vi "Inline Write (Interactions).vi"(8 "error in":errorcluster, 11 "RT State Variables in":T1 {"runtime data"."out object status BD"."Data Reference" format="%.0x"; "runtime data"."out object data BD"."Data Reference" format="%.0x"; "runtime data"."out interaction status BD"."Data Reference" format="%.0x"; "runtime data"."out interaction data BD"."Data Reference" format="%.0x"; "Settings"."objectData"."out object status BD"."Data Reference" format="%.0x"; "Settings"."objectData"."out object data BD"."Data Reference" format="%.0x"; "Settings"."objectData"."out interaction status BD"."Data Reference" format="%.0x"; "Settings"."objectData"."out interaction data BD"."Data Reference" format="%.0x"}) -> (0 "error out":errorcluster, 3 "RT State Variables out":T1 {"runtime data"."out object status BD"."Data Reference" format="%.0x"; "runtime data"."out object data BD"."Data Reference" format="%.0x"; "runtime data"."out interaction status BD"."Data Reference" format="%.0x"; "runtime data"."out interaction data BD"."Data Reference" format="%.0x"; "Settings"."objectData"."out object status BD"."Data Reference" format="%.0x"; "Settings"."objectData"."out object data BD"."Data Reference" format="%.0x"; "Settings"."objectData"."out interaction status BD"."Data Reference" format="%.0x"; "Settings"."objectData"."out interaction data BD"."Data Reference" format="%.0x"})   [LabVIEW 2019, in "HLA Custom Device Engine.lvlib"]
uses:
  HLA Custom Device Engine.lvlib
  RTStateVariables.ctl
  <vilib>/NI/NIVS Inline Async API/_VS Inline Async API/VS Inline Async API/VS Inline Async API.lvclass
  Shared/Compiled.Settings.ctl
  Shared/main_page_config.ctl
  Shared/object_managament_config.ctl
  Shared/interaction_parameter_configuration.ctl
  Shared/object_attribute_configuration.ctl
  Shared/object_status_info.ctl
  Shared/object_data.ctl
  <vilib>/NI VeriStand/Custom Device API/Block Data Reference.ctl
  <vilib>/NI VeriStand/Custom Device API/Data Reference.ctl
  RTruntimeData.ctl
  _typedefs/RThlaMapHelpers.ctl
  _typedefs/map_in_interaction.ctl
  _typedefs/map_interaction_value.ctl
  _typedefs/map_attr_param_data.ctl
  _typedefs/map_object.ctl
  _typedefs/map_object_key.ctl
  _typedefs/map_object_value.ctl
  _typedefs/map_object_instance.ctl
  _typedefs/map_object_instance_value.ctl
  _typedefs/map_object_vs_instance.ctl
  _typedefs/map_out_vs_ch_instanceId.ctl
  _typedefs/map_out_vs_ch_objects.ctl
  _typedefs/map_out_vs_ch_objects_value.ctl
  _typedefs/map_out_vs_ch_interactIonClass.ctl
  <vilib>/addons/hla/receiveInteractionEvent_type.ctl
  <vilib>/addons/hla/OrderType.ctl
  <vilib>/addons/hla/TransportationType.ctl
  <vilib>/addons/hla/reflectAttributeValuesEvent_type.ctl
  <vilib>/addons/hla/discoverObjectInstanceEvent_type.ctl
  <vilib>/addons/hla/removeObjectInstanceEvent_type.ctl
  <vilib>/NI VeriStand/Custom Device API/Global Data Refs.vi
  Data Encoding_Decoding/Set HLAfloat64BE.vi
  Data Encoding_Decoding/custom/Set fixed_coords.vi
  <vilib>/NI VeriStand/Custom Device API/Custom Device API.lvlib
  <vilib>/addons/hla/openrti_rti1516eLv.lvlib
  <vilib>/addons/hla/helpers/phvm.lvlib
  _Debug/VsDebugLibrary.lvlib
  Shared/HLA Custom Device Shared.lvlib
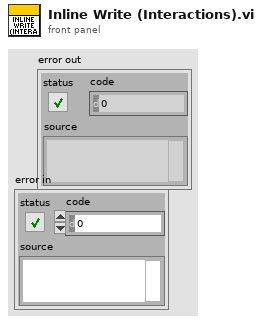
[diagram p1: front panel]
types:
  T1 = typedef "HLA Custom Device Engine.lvlib/RTStateVariables.ctl" = cluster{"Async":refnum<class "VS Inline Async API.lvclass">, "Settings":T2, "runtime data":T11}
  T2 = typedef "HLA Custom Device Shared.lvlib/Compiled.Settings.ctl" = cluster{"Name":string, "Async Init Timeout":u16, "main page properties":T3, "obiectConfig":T4, "objectStatus":T7, "objectData":T8}
  T3 = typedef "HLA Custom Device Shared.lvlib/main_page_config.ctl" = cluster{"Federate Execution Name":string, "Federate Type":string, "Local Designator Settings":string, "FOM Module":path, "mak mtl file":path, "FOM destination path":string, "MTL destination path":string}
  T4 = typedef "HLA Custom Device Shared.lvlib/object_managament_config.ctl" = cluster{"incoming interactions":T5[], "incoming objects":T6[], "outgoing interactions":T5[], "outgoing objects":T6[]}
  T5 = typedef "HLA Custom Device Shared.lvlib/interaction_parameter_configuration.ctl" = cluster{"interaction class name":string, "parameter name":string, "datatype":string, "vsChIndex":i32, "vsObjectId":string}
  T6 = typedef "HLA Custom Device Shared.lvlib/object_attribute_configuration.ctl" = cluster{"object class name":string, "instanceId":i32, "attribute name":string, "datatype":string, "vsChIndex":i32, "vsObjectId":string}
  T7 = typedef "HLA Custom Device Shared.lvlib/object_status_info.ctl" = cluster{"incoming interactions":map{string, map{string, i32}}, "incoming objects":map{string, map{string, i32}}, "outgoing interactions":map{string, map{string, i32}}, "outgoing objects":map{string, map{string, i32}}}
  T8 = typedef "HLA Custom Device Shared.lvlib/object_data.ctl" = cluster{"out interaction data BD":T9[], "out interaction data size":i32, "out interaction status BD":T9[], "out interaction status size":i32, "out object data BD":T9[], "out object data size":i32, "out object status BD":T9[], "out object status size":i32}
  T9 = typedef "Custom Device API.lvlib/Block Data Reference.ctl" = cluster{"Data Reference":T10, "Offset":u64, "Length":u64}
  T10 = typedef "Custom Device API.lvlib/Data Reference.ctl" = i32
  T11 = typedef "HLA Custom Device Engine.lvlib/RTruntimeData.ctl" = cluster{"rtiHandle":i64, "hlaMap":T12, "hla event registration":refnum<event-registration>, "out interaction data BD":T9[], "out interaction data":dbl[], "out interaction status BD":T9[], "out interaction status ":dbl[], "out object data BD":T9[], "out object data":dbl[], "out object status BD":T9[], "out object status ":dbl[]}
  T12 = typedef "HLA Custom Device Engine.lvlib/RThlaMapHelpers.ctl" = cluster{"in_interactionMap":T13, "in_objectMap":T16, "in_map_object_instance":T19, "in_map_vs_incoming_instance":T21, "out_map_vs_ch_instanceId":T22, "out_interactionMap":T13, "out_map_vs_ch_objectInstance":T23, "out_objectMap":T16, "out_map_vs_ch_interactionClass":T25}
  T13 = typedef "HLA Custom Device Engine.lvlib/map_in_interaction.ctl" = map{u64, T14}
  T14 = typedef "HLA Custom Device Engine.lvlib/map_interaction_value.ctl" = cluster{"infoChMap":map{string, i32}, "parameterMap":map{u64, T15}, "parHandleValueMap":u64}
  T15 = typedef "HLA Custom Device Engine.lvlib/map_attr_param_data.ctl" = cluster{"dataType":string, "offset":i32, "numOfElements":i32}
  T16 = typedef "HLA Custom Device Engine.lvlib/map_object.ctl" = map{T17, T18}
  T17 = typedef "HLA Custom Device Engine.lvlib/map_object_key.ctl" = cluster{"instanceId":i32, "objectClassHandle":u64}
  T18 = typedef "HLA Custom Device Engine.lvlib/map_object_value.ctl" = cluster{"infoChMap":map{string, i32}, "attributeMap":map{u64, T15}, "attrHandleSet":u64, "attrHandleValueMap":u64, "objectInstancePrefix":string}
  T19 = typedef "HLA Custom Device Engine.lvlib/map_object_instance.ctl" = map{u64, T20}
  T20 = typedef "HLA Custom Device Engine.lvlib/map_object_instance_value.ctl" = cluster{"objectClassHandle":u64, "objectInstanceName":string, "InstanceID":i32}
  T21 = typedef "HLA Custom Device Engine.lvlib/map_object_vs_instance.ctl" = map{u64, map{i32, u64}}
  T22 = typedef "HLA Custom Device Engine.lvlib/map_out_vs_ch_instanceId.ctl" = map{i32, i32}
  T23 = typedef "HLA Custom Device Engine.lvlib/map_out_vs_ch_objects.ctl" = map{i32, T24}
  T24 = typedef "HLA Custom Device Engine.lvlib/map_out_vs_ch_objects_value.ctl" = cluster{"objectInstanceHandle":u64, "objectClassHandle":u64}
  T25 = typedef "HLA Custom Device Engine.lvlib/map_out_vs_ch_interactIonClass.ctl" = map{i32, u64}
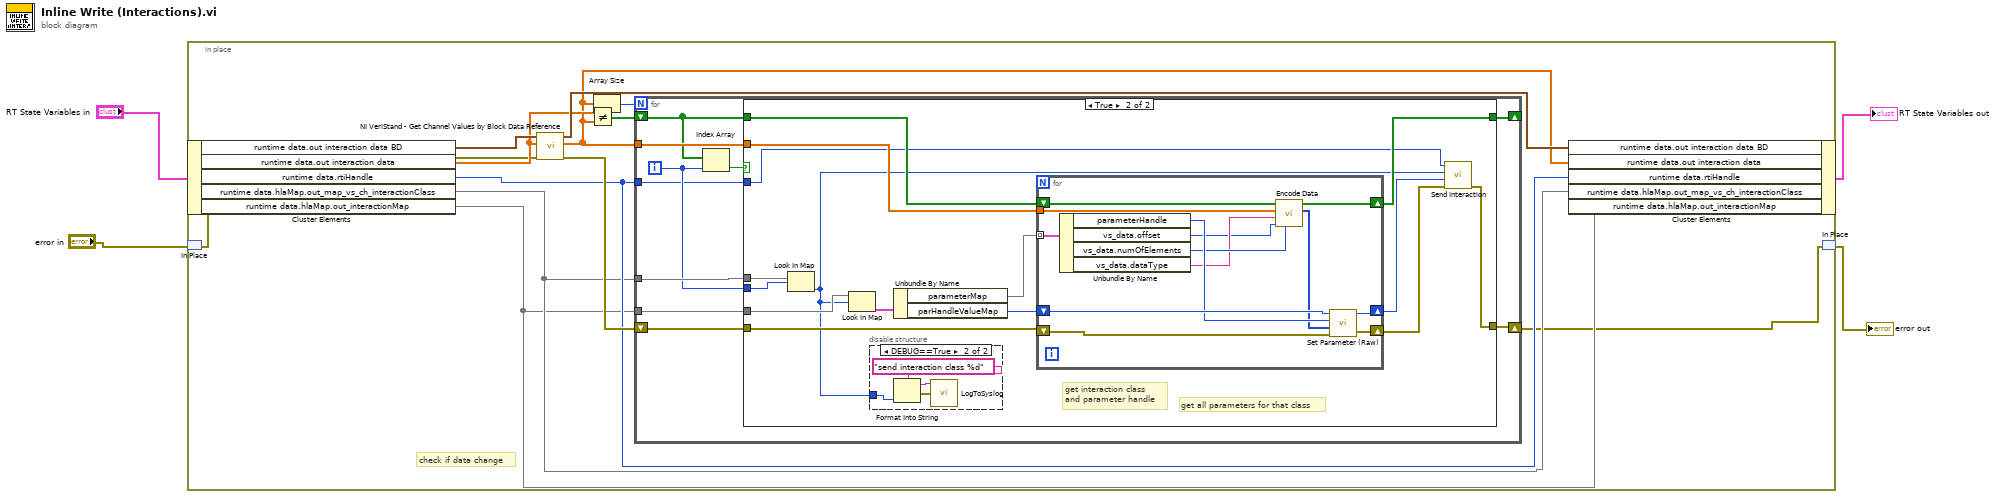
[diagram p0: block diagram]
diagram:
  n1 = in-place {
    # "check if data change"
    n2 = in-place-cluster #1("RT State Variables in") -> ("runtime data.out interaction data BD"=w16:T9[], "runtime data.out interaction data"=w8:dbl[], "runtime data.rtiHandle"=w11:i64, "runtime data.hlaMap.out_map_vs_ch_interactionClass"=w10:T25, "runtime data.hlaMap.out_interactionMap"=w9:T13)
    n3 = in-place-match #2("error in") -> (w6:errorcluster)
    n4 = call <vilib>:"NI VeriStand - Get Channel Values by Block Data Reference.vi"("error in (no error)"=w6, "Values Array in"=w8, "Block Data Ref"=w16) -> ("error out"=w14:errorcluster, "Values Array out"=w7:dbl[], "Block Data Ref dup"=w15:T9[])  [unwired: 6 in]
    n5 = Not Equal?(x=w8, y=w7) -> (x != y?=w13:bool[])
    n6 = Array Size(array=w7) -> (size(s)=w12:i32)
    n7 = for {
      N: w12 -> [_]
      tunnel: w10 -> [w25]
      tunnel: w9 -> [w24]
      tunnel: w7 -> [w22]
      shift-right: [w26] -> w5
      shift-left: w14 -> [w23]
      shift-right: [w18] -> _
      shift-left: w13 -> [w21]
      tunnel: w11 -> [w17]
      i -> [w19]
      n8 = Index Array(array=w21, index=w19) -> (element=w20:bool)
      n9 = case shown="True" w20 {
        tunnel: [w28 w43] -> w26
        tunnel: w25 -> [_ w42]
        tunnel: w24 -> [_ w41]
        tunnel: w23 -> [w28 w37]
        tunnel: w22 -> [_ w34]
        tunnel: w21 -> [w27 w33]
        tunnel: w19 -> [_ w30]
        tunnel: [w27 w32] -> w18
        tunnel: w17 -> [_ w31]
        frame False {
        }
        frame True {
          # "get all parameters for that class"
          # "get interaction class\nand parameter handle"
          n10 = Look In Map(map=w42, key=w30) -> (value=w29:u64)  [unwired: 1 in, 1 out]
          n11 = Look In Map(map=w41, key=w29) -> (value=w40:T14)  [unwired: 1 in, 1 out]
          n12 = disable-structure shown="DEBUG==True" {
            disable-tunnel: w29 -> [_ w44]
            frame condition #0 {
            }
            frame condition #1 (active) {
              n13 = Format Into String(format string="send interaction class %d", w44) -> (resulting string=w46:string, error out=w47:errorcluster)  [unwired: 2 in]
              n14 = call "LogToSyslog.vi"("error in (no error)"=w47, "message"=w46) -> ()  [unwired: 8 in, 2 out]
            }
          }
          n15 = Unbundle By Name(w40) -> ("parameterMap"=w38:map{u64, T15}, "parHandleValueMap"=w39:u64)
          n16 = for {
            shift-right: [w55] -> w35
            shift-left: w39 -> [w59]
            tunnel: w38 -> [w60] mode=indexing
            shift-right: [w57] -> w36
            shift-left: w37 -> [w58]
            tunnel: w34 -> [w51]
            shift-right: [w53] -> w32
            shift-left: w33 -> [w54]
            n17 = Unbundle By Name(w60) -> ("parameterHandle"=w56:u64, "vs_data.offset"=w48:i32, "vs_data.numOfElements"=w50:i32, "vs_data.dataType"=w49:string)
            n18 = call "Encode Data.vi"("numOfElements (1)"=w50, "offset"=w48, "dataType"=w49, "Values Array in"=w51, "changed flag array in"=w54) -> ("raw data out"=w52:u8[], "changed flag array out"=w53:bool[])  [unwired: 5 in]
            n19 = call <vilib>:"Set Parameter (Raw).vi"("error in"=w58, "data"=w52, "parameterHandle in"=w56, "parHandleValueMap in"=w59) -> ("error out"=w57:errorcluster, "parHandleValueMap out"=w55:u64)  [unwired: 5 in, 1 out]
          }
          n20 = call <vilib>:"Send Interaction.vi"("error in"=w36, "parHandleValueMap in"=w35, "interactionClassHandle in"=w29, "rtiHandle in"=w31) -> ("error out"=w43:errorcluster)  [unwired: 4 in, 3 out]
        }
      }
    }
    n21 = in-place-cluster #1("runtime data.out interaction data BD"=w15, "runtime data.out interaction data"=w7, "runtime data.rtiHandle"=w11, "runtime data.hlaMap.out_map_vs_ch_interactionClass"=w10, "runtime data.hlaMap.out_interactionMap"=w9) -> (→"RT State Variables out":T1)
    n22 = in-place-match #2(w5) -> (→"error out":errorcluster)
  }
